vi "Digital Reversed Order_Reversed Index.vi"(10 "radix":i32, 11 "length":i32) -> (0 "error":i32, 3 "Reversed Index":i32[](array[numeric]))   [LabVIEW 2020, in "NI_AAL_SignalOperation.lvlib"]
uses:
  <vilib>/Analysis/NI_AAL_SignalOperation.lvlib
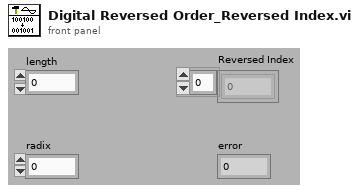
[diagram p1: front panel]
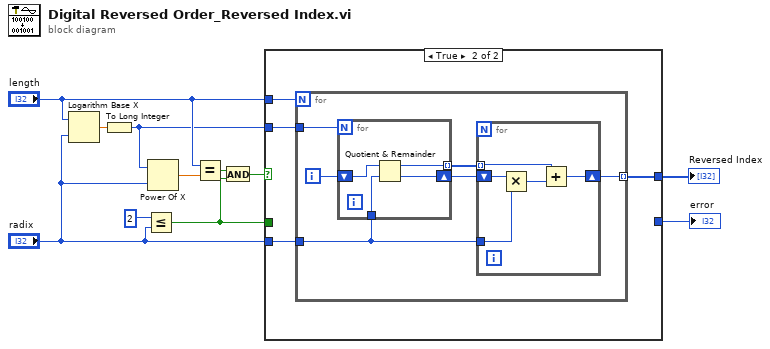
[diagram p0: block diagram]
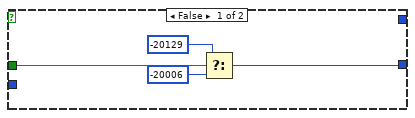
[diagram p2: hidden frame]
diagram:
  n1 = Logarithm Base X(1:"radix", 2:"length") -> (0:w11:dbl)
  n2 = To Long Integer(number=w11) -> (32bit integer=w7:i32)
  n3 = Less Or Equal?(x=2 ("y"), y="radix") -> (x <= y?=w4:bool)
  n4 = Power Of X(1:"radix", 2:w7) -> (0:w1:dbl)
  n5 = Equal?(x="length", y=w1) -> (x = y?=w10:bool)
  n6 = And(x=w10, y=w4) -> (x .and. y?=w9:bool)
  n7 = case shown="True" w9 {
    tunnel: "length" -> [_ w19]
    tunnel: "radix" -> [_ w18]
    tunnel: w7 -> [_ w17]
    tunnel: [_ w16] -> w6
    tunnel: w4 -> [w14 _]
    tunnel: [w13 _] -> w5
    frame False {
      n8 = Select(t=-20129, s=w14, f=-20006) -> (s? t:f=w13:i32)
    }
    frame True {
      n9 = for {
        N: w19 -> [_]
        tunnel: w18 -> [w21]
        tunnel: w17 -> [w25]
        tunnel: [w20] -> w16 mode=indexing
        i -> [w24]
        n10 = for {
          N: w25 -> [_]
          shift-right: [w32] -> w23
          shift-left: w24 -> [w34]
          tunnel: w21 -> [w33]
          tunnel: [w31] -> w22 mode=indexing
          n11 = Quotient & Remainder(x=w34, y=w33) -> (x-y*floor(x/y)=w31:i32, floor(x/y)=w32:i32)
        }
        n12 = for {
          shift-right: [w28] -> w20
          shift-left: w23 -> [w29]
          tunnel: w22 -> [w26] mode=indexing
          tunnel: w21 -> [w30]
          n13 = Multiply(x=w29, y=w30) -> (x*y=w27:i32)
          n14 = Add(x=w26, y=w27) -> (x+y=w28:i32)
        }
      }
    }
  }
  "Reversed Index" <- w6
  "error" <- w5
